vi "0.-Introducción LabView.vi"() -> ()   [LabVIEW 2020]
panel:
  in  "stop":bool
  out "resultado":dbl
  in  "y":dbl
  in  "x":dbl
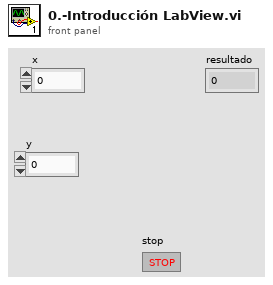
[diagram p1: front panel]
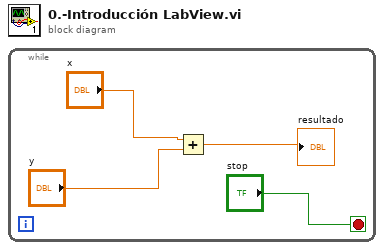
[diagram p0: block diagram]
diagram:
  n1 = while {
    stop <- "stop" stop-if-true
    n2 = Add(x="x", y="y") -> (x+y=→"resultado":dbl)
  }
